vi "unbuild waveform array_5.vi"(10 "Array":waveform(dbl)[](array[waveform])) -> (0 "l4":dbl, 1 "l3":dbl, 2 "l2":dbl, 3 "l1":dbl, 4 "t":dbl)   [LabVIEW 2014]
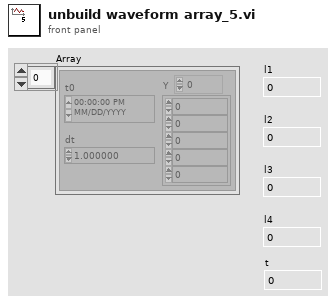
[diagram p1: front panel]
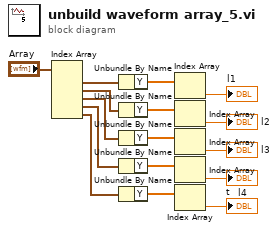
[diagram p0: block diagram]
diagram:
  n1 = Index Array(array="Array") -> (element #1=w2:waveform(dbl), element #2=w3:waveform(dbl), element #3=w4:waveform(dbl), element #4=w5:waveform(dbl), element #5=w6:waveform(dbl))  [unwired: 5 in]
  n2 = Unbundle By Name(w2) -> ("Y"=w7:dbl[])
  n3 = Unbundle By Name(w3) -> ("Y"=w10:dbl[])
  n4 = Unbundle By Name(w4) -> ("Y"=w11:dbl[])
  n5 = Unbundle By Name(w5) -> ("Y"=w12:dbl[])
  n6 = Unbundle By Name(w6) -> ("Y"=w9:dbl[])
  n7 = Index Array(array=w7) -> (element=→"l1":dbl)  [unwired: 1 in]
  n8 = Index Array(array=w10) -> (element=→"l2":dbl)  [unwired: 1 in]
  n9 = Index Array(array=w11) -> (element=→"l3":dbl)  [unwired: 1 in]
  n10 = Index Array(array=w12) -> (element=→"l4":dbl)  [unwired: 1 in]
  n11 = Index Array(array=w9) -> (element=→"t":dbl)  [unwired: 1 in]
